vi "Disactivate_Frames_Until_Get_Tracking_Results-1.vi"(6 "Delete Tracs Ref":refnum<vi>, 7 "Save pictures Ref":refnum<vi>, 8 "error IN":errorcluster, 9 "Frame Ref":refnum<vi>, 10 "Saved #  Ref":refnum<vi>, 11 "Raw # Ref":refnum<vi>) -> ()   [LabVIEW 2013]
doc: "Handling of buttons properties"
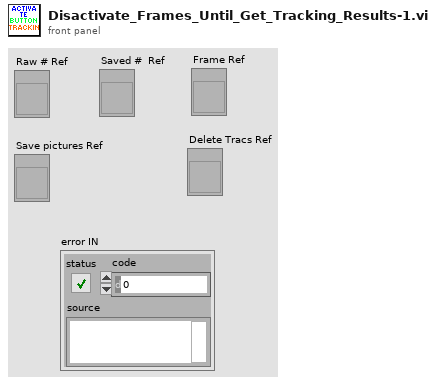
[diagram p1: front panel]
types:
  T1 = enum8{"Enabled", "Disabled", "Disabled and Grayed Out"}
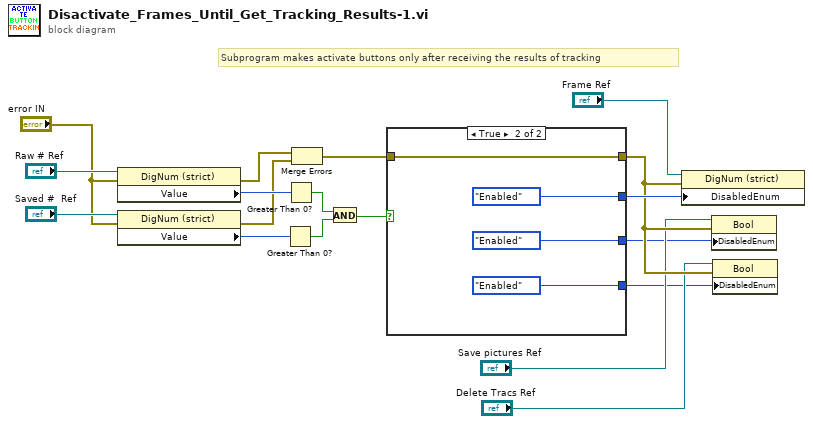
[diagram p0: block diagram]
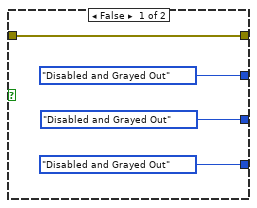
[diagram p2: hidden frame]
diagram:
  # "Subprogram makes activate buttons only after receiving the results of tracking"
  n1 = property on="Property Node" class="DigNum (strict)"(reference="Raw # Ref", error in="error IN") -> (error out=w10:errorcluster, "Value"=w16:i32)  [unwired: 1 out]
  n2 = property on="Property Node" class="DigNum (strict)"(reference="Saved #  Ref", error in="error IN") -> (error out=w9:errorcluster, "Value"=w14:i32)  [unwired: 1 out]
  n3 = Greater Than 0?(x=w14) -> (x > 0?=w12:bool)
  n4 = Greater Than 0?(x=w16) -> (x > 0?=w13:bool)
  n5 = Merge Errors(w10, w9) -> (w8:errorcluster)
  n6 = And(x=w13, y=w12) -> (x .and. y?=w11:bool)
  n7 = case shown="True" w11 {
    tunnel: w8 -> [w22 w26]
    tunnel: [w22 w26] -> w6
    tunnel: [T1."Disabled and Grayed Out" ("Disabled") T1."Enabled" ("Disabled")] -> w7
    tunnel: [T1."Disabled and Grayed Out" ("Disabled") T1."Enabled" ("Disabled")] -> w2
    tunnel: [T1."Disabled and Grayed Out" ("Disabled") T1."Enabled" ("Disabled")] -> w1
    frame False {
    }
    frame True {
    }
  }
  n8 = property on="Property Node" class="DigNum (strict)"(reference="Frame Ref", error in=w6, "DisabledEnum"=w7) -> ()  [unwired: 2 out]
  n9 = property on="Property Node" class="Bool"(reference="Save pictures Ref", error in=w6, "DisabledEnum"=w2) -> ()  [unwired: 2 out]
  n10 = property on="Property Node" class="Bool"(reference="Delete Tracs Ref", error in=w6, "DisabledEnum"=w1) -> ()  [unwired: 2 out]
